vi "Status.vi"(0 "VISA resource name":refnum<visa-resource-name>, 11 "error in (no error)":errorcluster, 12 "Output Loop":u16(ring)=2 items=["1"=1, "2"=2]) -> (1 "Setpoint Status":dbl format="%.4f", 2 "Heater Status":u16(ring) items=["Off", "Low (On)", "Medium", "High"], 3 "Heater Output %":dbl format="%.1f", 4 "VISA resource name out":refnum<visa-resource-name>, 13 "Ramping On?":bool, 14 "Ramping Active?":bool, 15 "error out":errorcluster)   [LabVIEW 2024]
uses:
  <instrlib>/Lake Shore 336/Lake Shore 336.lvlib
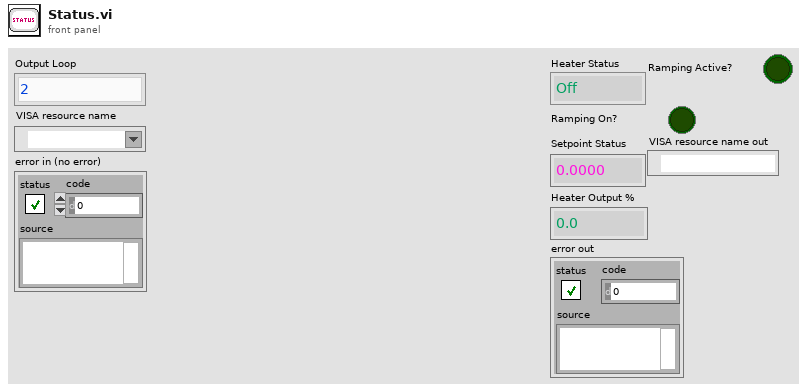
[diagram p1: front panel]
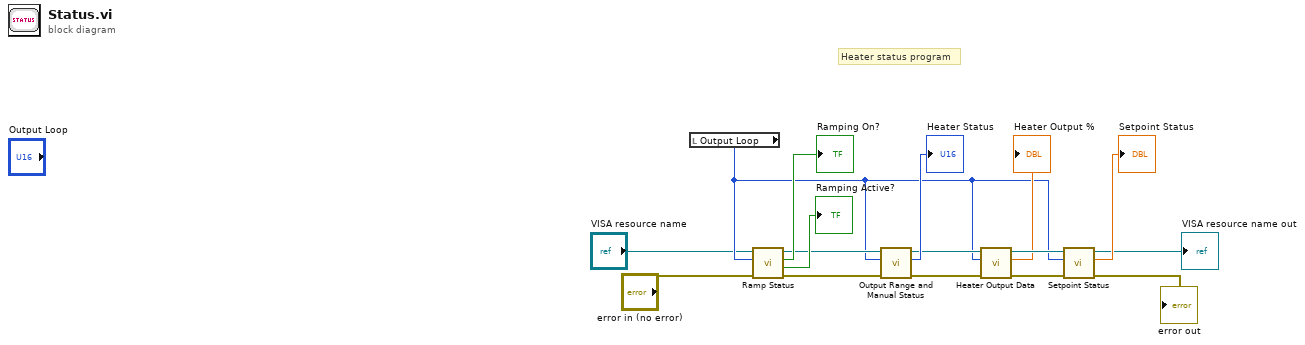
[diagram p0: block diagram]
diagram:
  # "Heater status program"
  n1 = local read "Output Loop"() -> (w5:u16)
  n2 = call <instrlib>:"Ramp Status.vi"("error in (no error)"="error in (no error)", "Output's Control Loop (1:1)"=w5, "VISA resource name"="VISA resource name") -> ("error out"=w11:errorcluster, "Ramping Active?"=→"Ramping Active?":bool, "Ramping On?"=→"Ramping On?":bool, "VISA resource name out"=w12:refnum<visa-resource-name>)  [unwired: 4 in, 1 out]
  n3 = call <instrlib>:"Output Range and Manual Status.vi"("error in (no error)"=w11, "Output (1:1)"=w5, "VISA resource name"=w12) -> ("error out"=w8:errorcluster, "Range (0:Off)"=→"Heater Status":u16, "VISA resource name out"=w10:refnum<visa-resource-name>)  [unwired: 5 in, 1 out]
  n4 = call <instrlib>:"Heater Output Data.vi"("error in (no error)"=w8, "Heater Output (1:1)"=w5, "VISA resource name"=w10) -> ("error out"=w7:errorcluster, "Output Value"=→"Heater Output %":dbl, "VISA resource name out"=w9:refnum<visa-resource-name>)  [unwired: 6 in]
  n5 = call <instrlib>:"Setpoint Status.vi"("error in (no error)"=w7, "Output (1:1)"=w5, "VISA resource name"=w9) -> ("error out"=→"error out":errorcluster, "Setpoint"=→"Setpoint Status":dbl, "VISA resource name out"=→"VISA resource name out":refnum<visa-resource-name>)  [unwired: 6 in]
